vi "OpenPanel(SubVI).vi"(6 "String":string, 9 "State":T1(ring), 10 "Wait Until Done":bool, 11 "Auto Dispose Reference":bool) -> ()   [LabVIEW 2021]
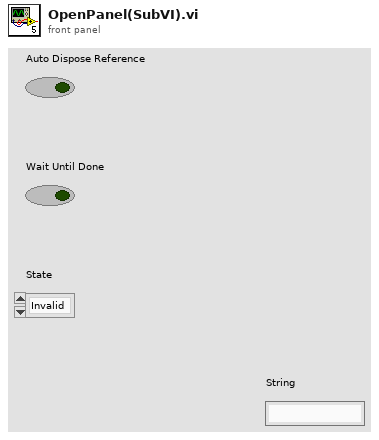
[diagram p1: front panel]
types:
  T1 = enum32{"Invalid", "Standard", "Closed", "Hidden", "Minimized", "Maximized"}
  T2 = enum32{"Bad", "Idle", "Run top level", "Running"}
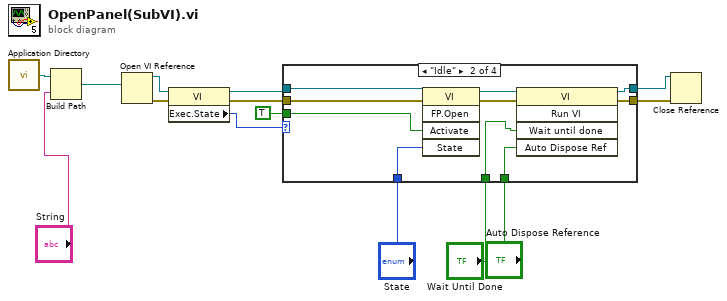
[diagram p0: block diagram]
diagram:
  n1 = call <vilib>:"Application Directory.vi"() -> ("Application Directory"=w2:path)
  n2 = Build Path(base path=w2, name or relative path="String") -> (appended path=w3:path)
  n3 = Open VI Reference(vi path=w3) -> (vi reference=w5:refnum<vi>, error out=w6:errorcluster)  [unwired: 5 in]
  n4 = property class="VI"(reference=w5, error in=w6) -> (reference out=w8:refnum<vi>, error out=w9:errorcluster, "Exec.State"=w7:T2)
  n5 = case shown="\"Idle\"" w7 {
    tunnel: [w16 w24 w28 w30] -> w1
    tunnel: [w15 w23 w27 w29] -> w4
    tunnel: w8 -> [w16 w22 w28 w30]
    tunnel: w9 -> [w15 w21 w27 w29]
    tunnel: TRUE ("Conf button") -> [_ w20 _ _]
    tunnel: "Wait Until Done" -> [_ w19 _ _]
    tunnel: "Auto Dispose Reference" -> [_ w18 _ _]
    tunnel: "State" -> [_ w17 _ _]
    frame "Bad", Default {
    }
    frame "Idle" {
      n6 = invoke class="VI" method="FP.Open"(reference=w22, error in=w21, "Activate"=w20, "State"=w17) -> (reference out=w26:refnum<vi>, error out=w25:errorcluster)  [unwired: 1 in, 3 out]
      n7 = invoke class="VI" method="Run VI"(reference=w26, error in=w25, "Wait until done"=w19, "Auto Dispose Ref"=w18) -> (reference out=w24:refnum<vi>, error out=w23:errorcluster)  [unwired: 1 in, 3 out]
    }
    frame "Run top level" {
    }
    frame "Running" {
    }
  }
  n8 = Close Reference(reference=w1, error in (no error)=w4) -> ()  [unwired: 1 out]
